vi "GetDateTimeDBFormat.vi"() -> (0 "Time in 24h format, e.g. 13:40:54":string="%m", 3 "Abbreviated Date, e.g. 13 Nov 2020":string="%m")   [LabVIEW 2019]
panel:
  out "Minute":string="%m"
  out "Hour in 24h format":string="%m"
  out "Second":string="%m"
  out "Year Number":string="%m"
  out "Day Number":string="%m"
  out "Abbreviated Month Name \n(OS language independent)":string="%m"
  out "Month Number":string="%m"
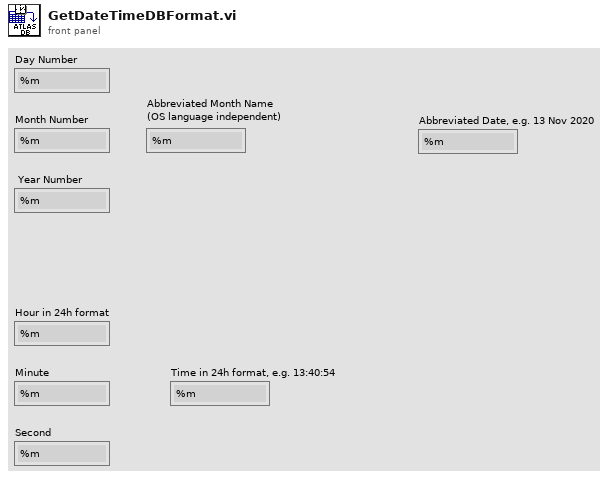
[diagram p1: front panel]
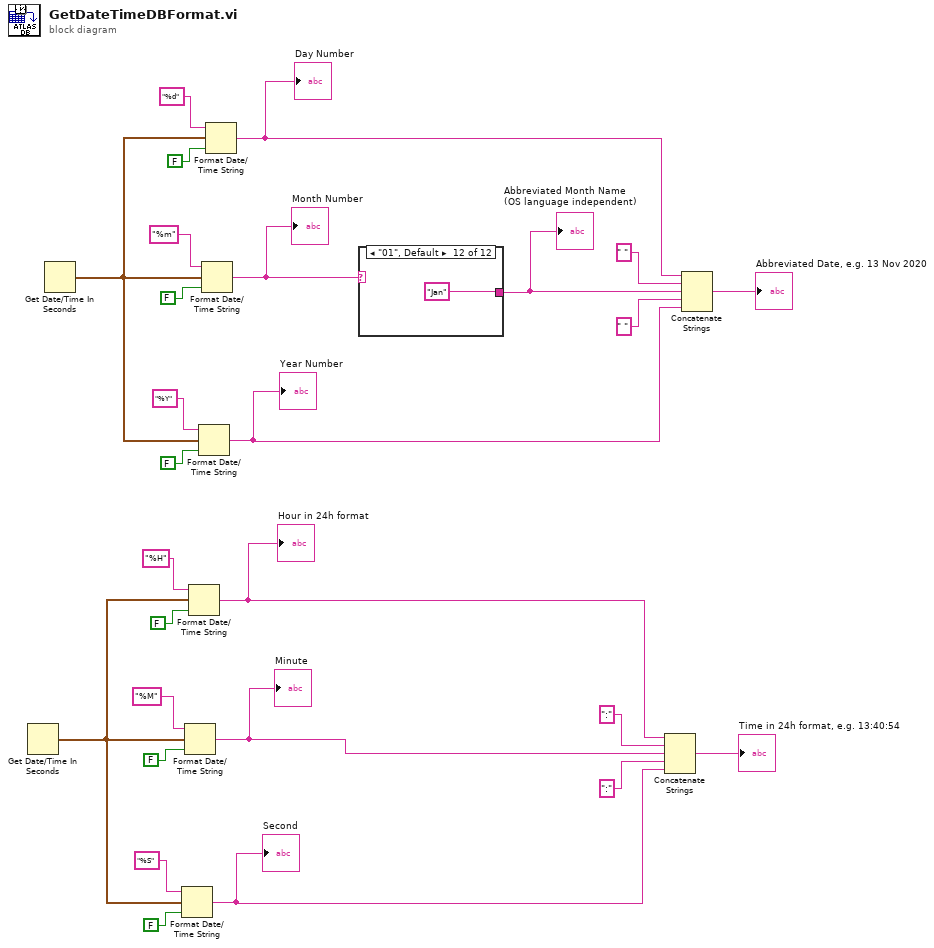
[diagram p0: block diagram]
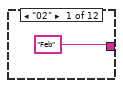
[diagram p2: hidden frame]
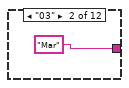
[diagram p3: hidden frame]
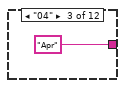
[diagram p4: hidden frame]
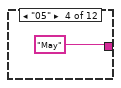
[diagram p5: hidden frame]
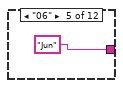
[diagram p6: hidden frame]
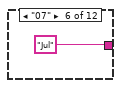
[diagram p7: hidden frame]
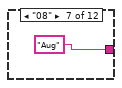
[diagram p8: hidden frame]
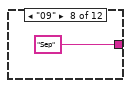
[diagram p9: hidden frame]
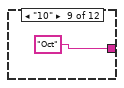
[diagram p10: hidden frame]
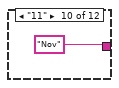
[diagram p11: hidden frame]
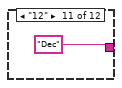
[diagram p12: hidden frame]
diagram:
  n1 = Get Date/Time In Seconds() -> (seconds since 1Jan1904=w8:timestamp)
  n2 = Get Date/Time In Seconds() -> (seconds since 1Jan1904=w20:timestamp)
  n3 = Format Date/Time String(time format string (%c)="%S", seconds (now)=w8, UTC format=FALSE) -> (date/time string=w10:string)
  "Second" <- w10
  n4 = Format Date/Time String(time format string (%c)="%M", seconds (now)=w8, UTC format=FALSE) -> (date/time string=w1:string)
  "Minute" <- w1
  n5 = Format Date/Time String(time format string (%c)="%H", seconds (now)=w8, UTC format=FALSE) -> (date/time string=w11:string)
  "Hour in 24h format" <- w11
  n6 = Format Date/Time String(time format string (%c)="%Y", seconds (now)=w20, UTC format=FALSE) -> (date/time string=w17:string)
  "Year Number" <- w17
  n7 = Format Date/Time String(time format string (%c)="%m", seconds (now)=w20, UTC format=FALSE) -> (date/time string=w26:string)
  "Month Number" <- w26
  n8 = Format Date/Time String(time format string (%c)="%d", seconds (now)=w20, UTC format=FALSE) -> (date/time string=w16:string)
  "Day Number" <- w16
  n9 = case shown="\"01\", Default" w26 {
    tunnel: ["Feb" "Mar" "Apr" "May" "Jun" "Jul" "Aug" "Sep" "Oct" "Nov" "Dec" "Jan"] -> w18
    frame "02" {
    }
    frame "03" {
    }
    frame "04" {
    }
    frame "05" {
    }
    frame "06" {
    }
    frame "07" {
    }
    frame "08" {
    }
    frame "09" {
    }
    frame "10" {
    }
    frame "11" {
    }
    frame "12" {
    }
    frame "01", Default {
    }
  }
  "Abbreviated Month Name \n(OS language independent)" <- w18
  n10 = Concatenate Strings(w11, ":", w1, ":", w10) -> (→"Time in 24h format, e.g. 13:40:54":string)
  n11 = Concatenate Strings(w16, " ", w18, " ", w17) -> (→"Abbreviated Date, e.g. 13 Nov 2020":string)
